vi "GAME OVER.vi"(0 "stop":bool, 1 "name":string) -> ()   [LabVIEW 2014]
uses:
  gameover.ctl
  gameover2.ctl
panel:
  out "concatenated string":T1
  out "String":T2="GAME OVER"
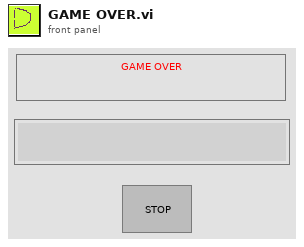
[diagram p1: front panel]
types:
  T1 = typedef "gameover2.ctl" = string
  T2 = typedef "gameover.ctl" = string
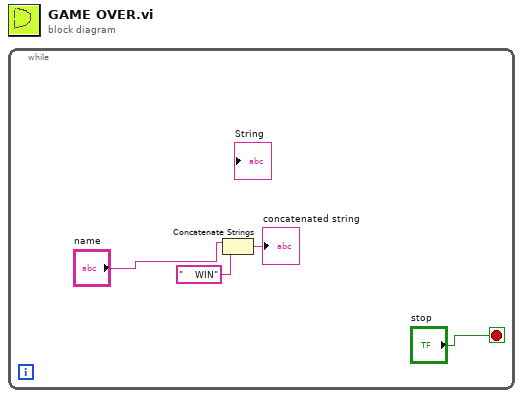
[diagram p0: block diagram]
diagram:
  n1 = while {
    stop <- "stop" stop-if-true
    n2 = Concatenate Strings("name", "    WIN" ("string")) -> (→"concatenated string":string)
  }
